vi "Add Pulse Recorder.vi"(6 "Reset":bool, 8 "error in (no error)":errorcluster, 9 "Auto launch":bool=TRUE, 10 "Module type":T1, 11 "Monitor-Pulse in":refnum<class "Monitor-Pulse.lvclass">) -> (0 "error out":errorcluster, 3 "Monitor-Pulse out":refnum<class "Monitor-Pulse.lvclass">)   [LabVIEW 2016, in "Monitor-Pulse.lvclass"]
uses:
  Monitor-Pulse.lvclass
  Controllers/Application Controller/Module Types.ctl
  Monitor-Pulse.lvclass/Monitor-Pulse.ctl
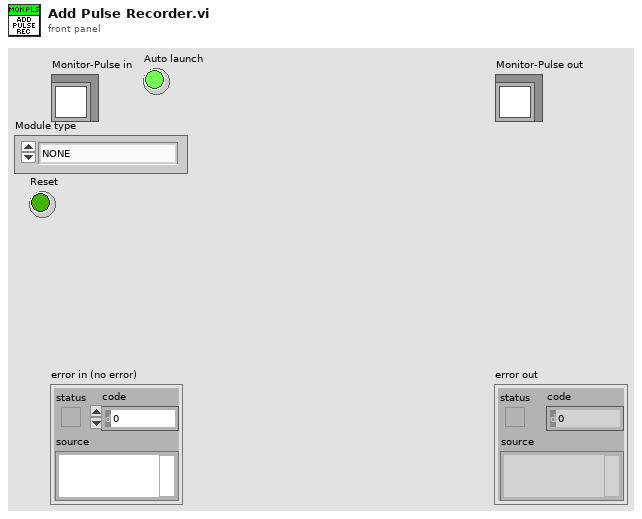
[diagram p1: front panel]
types:
  T1 = typedef "Module Types.ctl" = enum16{"NONE", "NI-DAQmx", "NI-Scope", "Red Pitaya Digitizer", "GaGe", "VISA Device", "Red Pitaya Lockin", "Monitor Controller", "Pulse Controller", "Integrate Pulse", "Lockin Processor", "File converter", "NHMFL Synthesizer", "Micron Hyperion", "Spectrum Recorder", "Resonance Detector", "TCP Communications", "Format Resonances"}
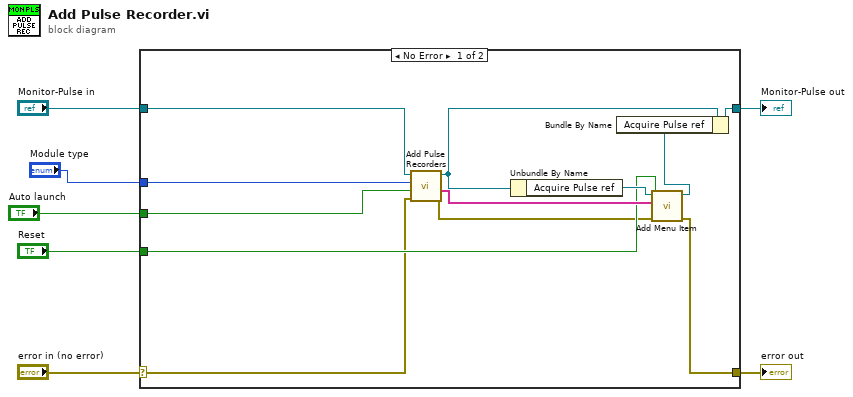
[diagram p0: block diagram]
diagram:
  n1 = case shown="No Error" "error in (no error)" {
    selector: "error in (no error)" -> [w9 w21]
    tunnel: [w8 w21] -> w6
    tunnel: [w11 w20] -> w4
    tunnel: "Monitor-Pulse in" -> [w19 w20]
    tunnel: "Module type" -> [w18 _]
    tunnel: "Auto launch" -> [w17 _]
    tunnel: "Reset" -> [w13 _]
    frame No Error {
      n2 = call-dynamic "Add Pulse Recorders.vi"("error in (no error)"=w9, "Auto launch"=w17, "Module type"=w18, "Monitor-Pulse in"=w19) -> ("error out"=w12:errorcluster, "Actor names out"=w14:string[], "Monitor-Pulse out"=w16:refnum<class "Monitor-Pulse.lvclass">)  [unwired: 4 in, 1 out]
      n3 = Unbundle By Name(w16) -> ("Acquire Pulse ref"=w15:refnum<vi>)
      n4 = call "Add Menu Item.vi"("error in (no error)"=w12, "Reset"=w13, "Item Names"=w14, "Queed Listbox ref"=w15) -> ("error out"=w8:errorcluster, "Queed Listbox ref out"=w10:refnum<vi>)  [unwired: 5 in, 1 out]
      n5 = Bundle By Name(cluster=w16, "Acquire Pulse ref"=w10) -> (w11:refnum<class "Monitor-Pulse.lvclass">)
    }
    frame Error {
    }
  }
  "error out" <- w6
  "Monitor-Pulse out" <- w4
